vi "get last calibration.vi"(8 "error in (no error)":errorcluster caption="Fehler (Eingang, kein Fehler)", 11 "Device (Eingang)":refnum<class "Device.lvclass">) -> (0 "error out":errorcluster caption="Fehler (Ausgang)", 2 "last calibration":string, 3 "Device (Ausgang)":refnum<class "Device.lvclass">)   [LabVIEW 2013, in "DatenKlassen.lvlib" / "Device.lvclass"]
uses:
  Device.lvclass
  Device.lvclass/Device.ctl
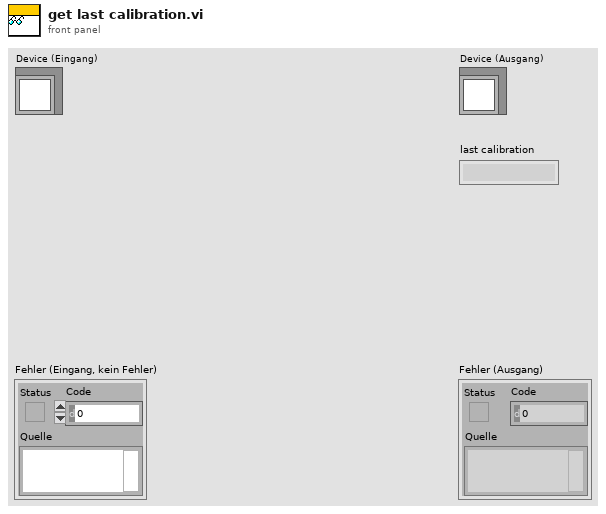
[diagram p1: front panel]
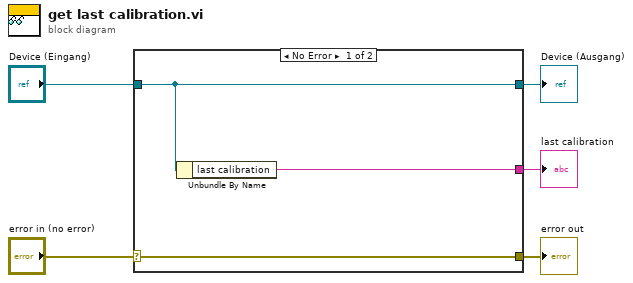
[diagram p0: block diagram]
diagram:
  n1 = case shown="No Error" "error in (no error)" {
    selector: "error in (no error)" -> [w8 w9]
    tunnel: [w8 w9] -> w4
    tunnel: [w7 w10] -> w2
    tunnel: "Device (Eingang)" -> [w7 w10]
    tunnel: [w6 _] -> w1
    frame No Error {
      n2 = Unbundle By Name(w7) -> ("last calibration"=w6:string)
    }
    frame Error {
    }
  }
  "error out" <- w4
  "Device (Ausgang)" <- w2
  "last calibration" <- w1
